vi "VISA_Test.vi"() -> ()   [LabVIEW 2016]
uses:
  <vilib>/Instr/_visa.llb/VISA Configure Serial Port (Instr).vi
panel:
  out "find list":string[](array[string])=["ASRL1::INSTR", "ASRL2::INSTR", "ASRL10::INSTR"]
  out "error out":errorcluster
  in  "VISA resource name":refnum<visa-resource-name>="ASRL1::INSTR"
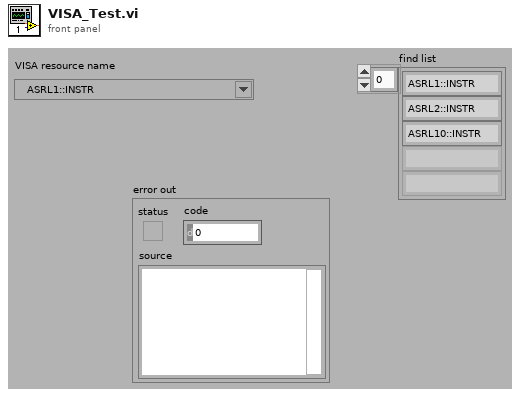
[diagram p1: front panel]
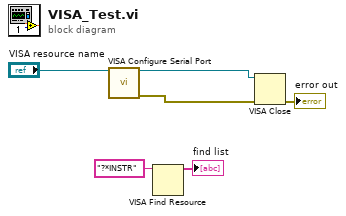
[diagram p0: block diagram]
diagram:
  n1 = call-poly "VISA Configure Serial Port"("VISA resource name"="VISA resource name") -> ("VISA resource name out"=w5:refnum<visa-resource-name>, "error out"=w4:errorcluster)  [unwired: 13 in]
  n2 = VISA Find Resource(11:"?*INSTR" ("expression (\"?*\")")) -> (3:→"find list":string[])  [unwired: 2 in, 2 out]
  n3 = VISA Close(VISA resource name=w5, error in (no error)=w4) -> (error out=→"error out":errorcluster)
